vi "XML - Remove System Mapping.vi"(8 "error in (no error)":errorcluster, 10 "Channel Path Destination":string, 11 "Item Ref in":T1 format="%.0x") -> (0 "error out":errorcluster, 3 "Item Ref out":T1 format="%.0x")   [LabVIEW 2019, in "UDP-Custom-Device System Explorer.lvlib"]
uses:
  UDP-Custom-Device System Explorer.lvlib
  <vilib>/NI VeriStand/Custom Device API/Custom Device Item Ref.ctl
  NationalInstruments.VeriStand.SystemDefinitionAPI
  <vilib>/NI VeriStand/Custom Device API/Custom Device API.lvlib
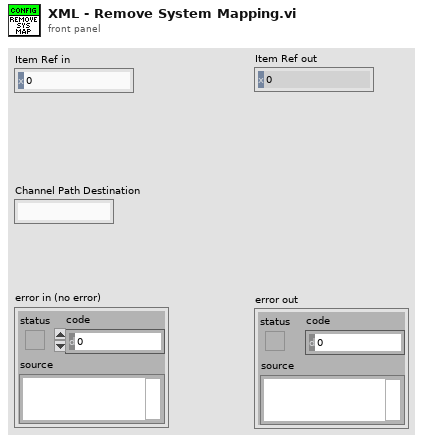
[diagram p1: front panel]
types:
  T1 = typedef "Custom Device API.lvlib/Custom Device Item Ref.ctl" = u64
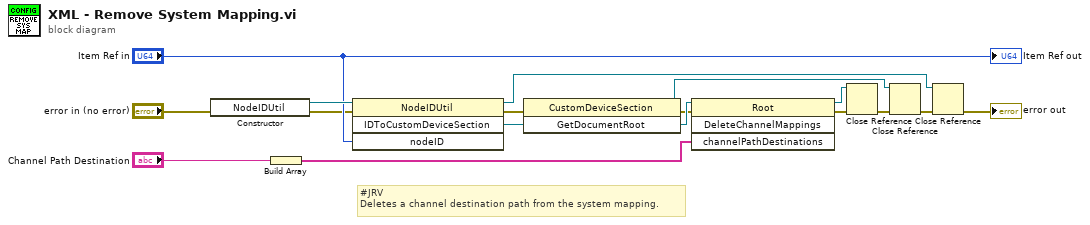
[diagram p0: block diagram]
diagram:
  # "#JRV\nDeletes a channel destination path from the system mapping."
  n1 = constructor class="NodeIDUtil"(error in="error in (no error)") -> (reference out=w10:refnum<k24>, error out=w5:errorcluster)  [unwired: 2 in, 1 out]
  n2 = Build Array("Channel Path Destination") -> (w8:string[])
  n3 = invoke class="NodeIDUtil" method="IDToCustomDeviceSection"(reference=w10, error in=w5, "nodeID"="Item Ref in") -> (reference out=w17:refnum<k24>, error out=w4:errorcluster, "IDToCustomDeviceSection"=w11:refnum<k24>)  [unwired: 1 in, 1 out]
  n4 = invoke class="CustomDeviceSection" method="GetDocumentRoot"(reference=w11, error in=w4) -> (reference out=w15:refnum<k24>, error out=w3:errorcluster, "GetDocumentRoot"=w12:refnum<k24>)  [unwired: 1 in]
  n5 = invoke class="Root" method="DeleteChannelMappings"(reference=w12, error in=w3, "channelPathDestinations"=w8) -> (reference out=w13:refnum<k24>, error out=w2:errorcluster)  [unwired: 1 in, 2 out]
  n6 = Close Reference(reference=w13, error in (no error)=w2) -> (error out=w14:errorcluster)
  n7 = Close Reference(reference=w15, error in (no error)=w14) -> (error out=w16:errorcluster)
  n8 = Close Reference(reference=w17, error in (no error)=w16) -> (error out=→"error out":errorcluster)
  "Item Ref out" <- "Item Ref in"
